vi "HornScanAbort_Recipe_with_HornScan_SUB_VI.vi"(0 "connection ID":refnum<k5>, 2 "Receipe Msg ID":u32, 3 "Receipe Message length":u32, 4 "Response ID":i32, 5 "error in (no error)":errorcluster, 8 "Start Frequency":u32, 9 "Time Delay":u16, 10 "Stop Frequency":u32, 11 "Max Amplitude":u16, 12 "Frequency Step":u16, 13 "Max Current":u16) -> (14 "Pass":string="Horn Scan Success", 15 "connection ID_out":refnum<k5>, 17 "Abort result":string="Horn Scan Success", 19 "error out":errorcluster)   [LabVIEW 2017]
panel:
  in  "SetDigitalTuneWithHornScan":u16
  # "OUTPUT"
  # "INPUT"
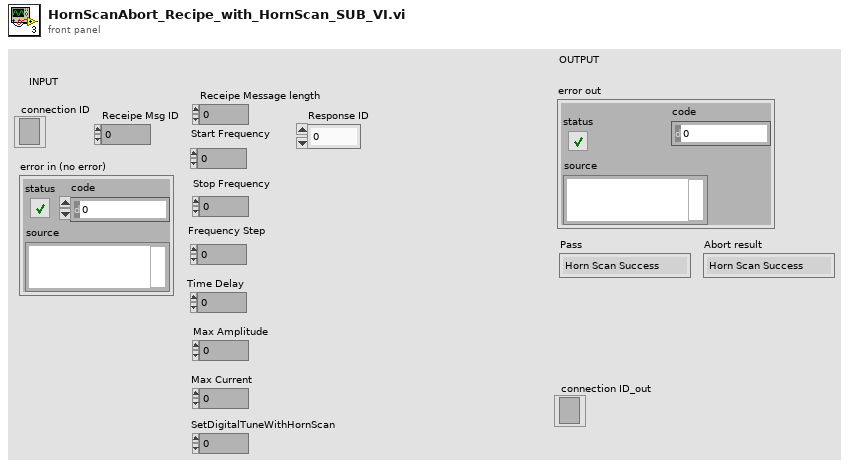
[diagram p1: front panel]
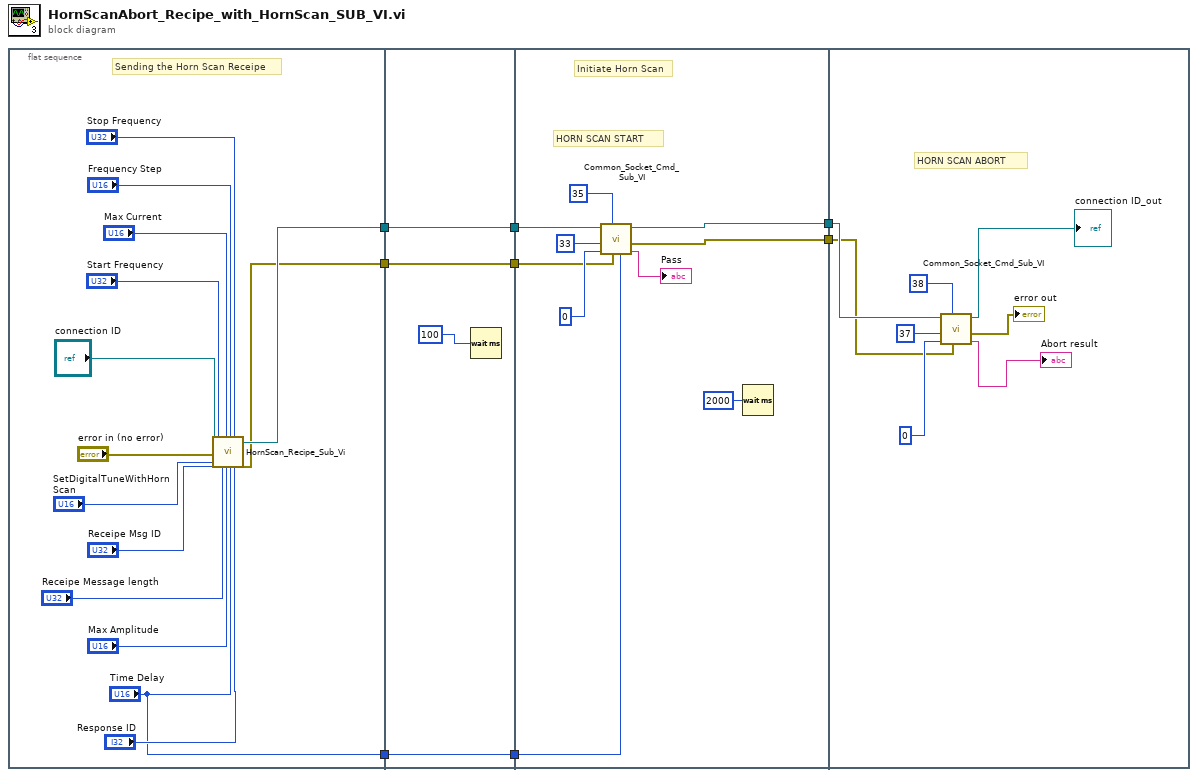
[diagram p0: block diagram]
diagram:
  n1 = flat-sequence {
    tunnel: [w13] -> w8
    tunnel: [w12] -> w5
    tunnel: ["Time Delay"] -> w4
    tunnel: w8 -> [w26]
    tunnel: [w26] -> w7
    tunnel: [w25] -> w6
    tunnel: w5 -> [w25]
    tunnel: w4 -> [w23]
    tunnel: [w23] -> w3
    tunnel: w7 -> [w36]
    tunnel: w6 -> [w33]
    tunnel: [w30] -> w2
    tunnel: [w29] -> w1
    tunnel: w3 -> [w28]
    tunnel: w2 -> [w41]
    tunnel: w1 -> [w40]
    frame #0 {
      # "Sending the Horn Scan Receipe"
      n2 = call "HornScan_Recipe_Sub_Vi.vi"("connection ID"="connection ID", "error in (no error)"="error in (no error)", "SetDigitalTuneWithHornScan"="SetDigitalTuneWithHornScan", "Receipe Msg ID"="Receipe Msg ID", "Start Frequency"="Start Frequency", "Receipe Message length"="Receipe Message length", "Max Current"="Max Current", "Max Amplitude"="Max Amplitude", "Frequency Step"="Frequency Step", "Time Delay"="Time Delay", "Stop Frequency"="Stop Frequency", "Response ID"="Response ID") -> ("connection ID"=w13:refnum<k5>, "error out"=w12:errorcluster)  [unwired: 13 in, 1 out]
    }
    frame #1 {
      n3 = Wait (ms)(milliseconds to wait=u32 100) -> ()  [unwired: 1 out]
    }
    frame #2 {
      # "HORN SCAN START"
      # "Initiate Horn Scan"
      n4 = call "Common_Socket_Cmd_Sub_VI.vi"("Time Delay"=w28, "Common Socket Error in"=w33, "Response ID 1"=u8 35, "Operation Message Length 1"=0, "Operation Message ID 1"=33, "connection ID"=w36) -> ("Status"=→"Pass":string, "error out"=w29:errorcluster, "connection ID"=w30:refnum<k5>)  [unwired: 3 in]
      n5 = Wait (ms)(milliseconds to wait=u32 2000) -> ()  [unwired: 1 out]
    }
    frame #3 {
      # "HORN SCAN ABORT"
      n6 = call "Common_Socket_Cmd_Sub_VI.vi"("Common Socket Error in"=w40, "Response ID 1"=u8 38, "Operation Message Length 1"=0, "Operation Message ID 1"=37, "connection ID"=w41) -> ("Status"=→"Abort result":string, "error out"=→"error out":errorcluster, "connection ID"=→"connection ID_out":refnum<k5>)  [unwired: 4 in]
    }
  }
